vi "McPhersonScan.vi"   [LabVIEW 2019]
types:
  T1 = enum16{"_Quit_", "Init", "Idle", "Error", "BeginScan", "SlewToZ1", "SlewPause", "StartScan", "Scanning", "ScanPause", "FinishScan", "Quit", "BeginSlew", "ResetBacklash"}
  T2 = enum16{"-Slew", "ScanN or SlewN or (Z0=Z1 & FinishScan)", "Error", "Z0=Z1 & BeginScan", "PauseY", "default"}
  T3 = enum16{"ScanN", "Error", "PassZ2", "PauseY", "default"}
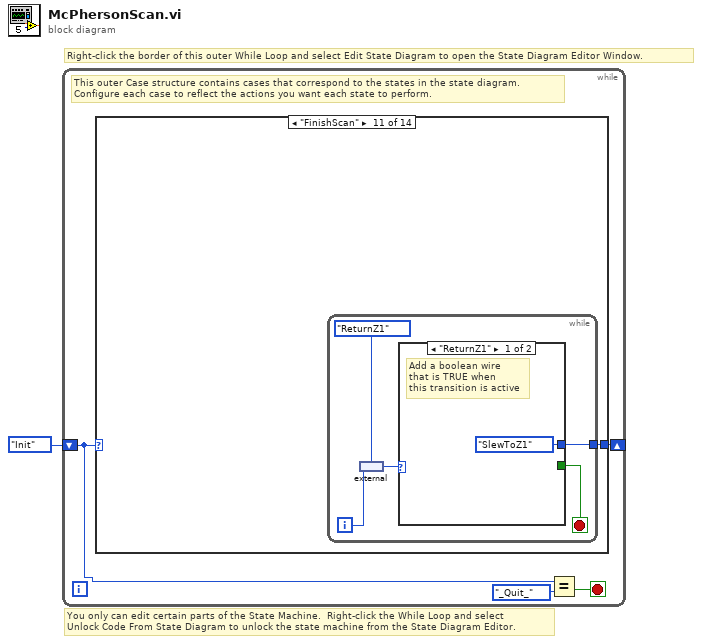
[diagram p0: block diagram]
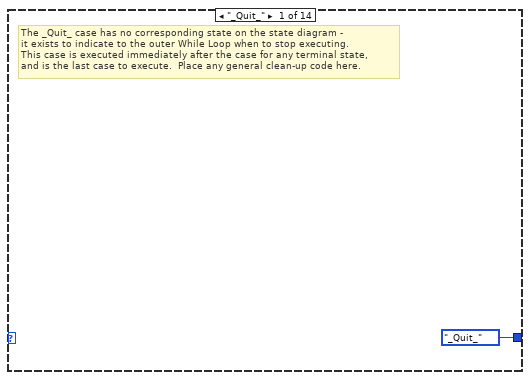
[diagram p2: hidden frame]
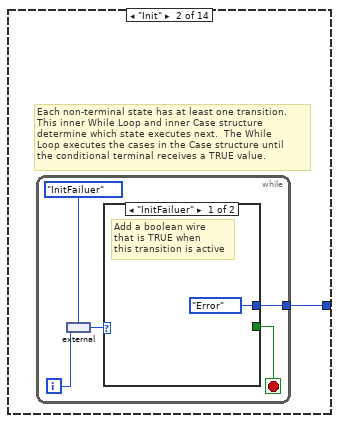
[diagram p3: hidden frame]
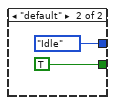
[diagram p4: hidden frame]
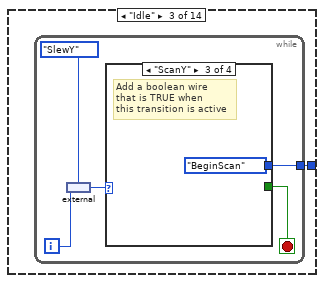
[diagram p5: hidden frame]
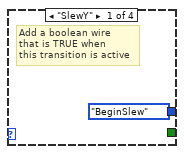
[diagram p6: hidden frame]
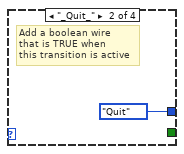
[diagram p7: hidden frame]
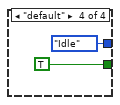
[diagram p8: hidden frame]
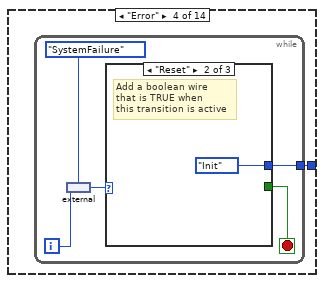
[diagram p9: hidden frame]
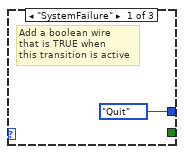
[diagram p10: hidden frame]
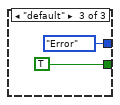
[diagram p11: hidden frame]
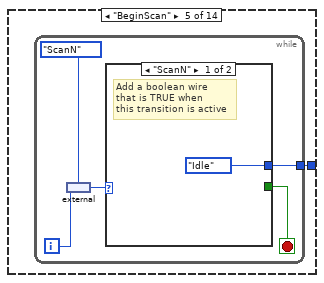
[diagram p12: hidden frame]
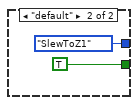
[diagram p13: hidden frame]
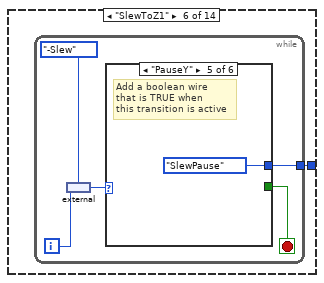
[diagram p14: hidden frame]
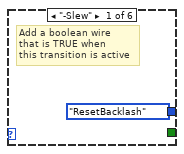
[diagram p15: hidden frame]
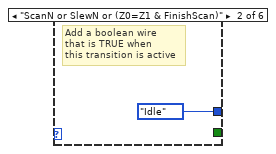
[diagram p16: hidden frame]
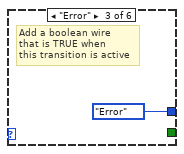
[diagram p17: hidden frame]
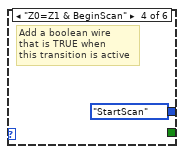
[diagram p18: hidden frame]
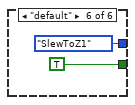
[diagram p19: hidden frame]
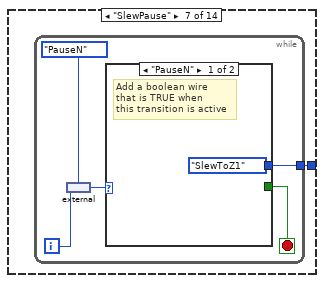
[diagram p20: hidden frame]
diagram:
  # "Right-click the border of this outer While Loop and select Edit State Diagram to open the State Diagram Editor Window."
  # "You only can edit certain parts of the State Machine.  Right-click the While Loop and select \nUnlock Code From State Diagram to unlock the state machine from the State Diagram Editor."
  n1 = while {
    shift-right: [w4] -> _
    shift-left: T1."Init" -> [w5]
    stop <- w3 stop-if-true
    # "This outer Case structure contains cases that correspond to the states in the state diagram.  \nConfigure each case to reflect the actions you want each state to perform."
    n2 = case shown="\"FinishScan\"" w5 {
      tunnel: [T1."_Quit_" w7 w21 w37 w52 w66 w84 w98 w111 w128 w142 w156 w169 w182] -> w4
      frame "_Quit_" {
        # "The _Quit_ case has no corresponding state on the state diagram -\nit exists to indicate to the outer While Loop when to stop executing.\nThis case is executed immediately after the case for any terminal state, \nand is the last case to execute.  Place any general clean-up code here."
      }
      frame "Init" {
        # "Each non-terminal state has at least one transition.\nThis inner While Loop and inner Case structure \ndetermine which state executes next.  The While \nLoop executes the cases in the Case structure until \nthe conditional terminal receives a TRUE value."
        n3 = while {
          tunnel: [w9] -> w7
          i -> [w12]
          stop <- w8 stop-if-true
          n4 = external(enum16{"InitFailuer", "default"}."InitFailuer", w12) -> (w10:enum16{"InitFailuer", "default"})
          n5 = case shown="\"InitFailuer\"" w10 {
            tunnel: [T1."Error" T1."Idle"] -> w9
            tunnel: [_ TRUE] -> w8
            frame "InitFailuer" {
              # "Add a boolean wire\nthat is TRUE when\nthis transition is active"
            }
            frame "default" {
            }
          }
        }
      }
      frame "Idle" {
        n6 = while {
          tunnel: [w23] -> w21
          i -> [w26]
          stop <- w22 stop-if-true
          n7 = external(enum16{"SlewY", "_Quit_", "ScanY", "default"}."SlewY", w26) -> (w24:enum16{"SlewY", "_Quit_", "ScanY", "default"})
          n8 = case shown="\"ScanY\"" w24 {
            tunnel: [T1."BeginSlew" T1."Quit" T1."BeginScan" T1."Idle"] -> w23
            tunnel: [_ _ _ TRUE] -> w22
            frame "SlewY" {
              # "Add a boolean wire\nthat is TRUE when\nthis transition is active"
            }
            frame "_Quit_" {
              # "Add a boolean wire\nthat is TRUE when\nthis transition is active"
            }
            frame "ScanY" {
              # "Add a boolean wire\nthat is TRUE when\nthis transition is active"
            }
            frame "default" {
            }
          }
        }
      }
      frame "Error" {
        n9 = while {
          tunnel: [w39] -> w37
          i -> [w42]
          stop <- w38 stop-if-true
          n10 = external(enum16{"SystemFailure", "Reset", "default"}."SystemFailure", w42) -> (w40:enum16{"SystemFailure", "Reset", "default"})
          n11 = case shown="\"Reset\"" w40 {
            tunnel: [T1."Quit" T1."Init" T1."Error"] -> w39
            tunnel: [_ _ TRUE] -> w38
            frame "SystemFailure" {
              # "Add a boolean wire\nthat is TRUE when\nthis transition is active"
            }
            frame "Reset" {
              # "Add a boolean wire\nthat is TRUE when\nthis transition is active"
            }
            frame "default" {
            }
          }
        }
      }
      frame "BeginScan" {
        n12 = while {
          tunnel: [w54] -> w52
          i -> [w57]
          stop <- w53 stop-if-true
          n13 = external(enum16{"ScanN", "default"}."ScanN", w57) -> (w55:enum16{"ScanN", "default"})
          n14 = case shown="\"ScanN\"" w55 {
            tunnel: [T1."Idle" T1."SlewToZ1"] -> w54
            tunnel: [_ TRUE] -> w53
            frame "ScanN" {
              # "Add a boolean wire\nthat is TRUE when\nthis transition is active"
            }
            frame "default" {
            }
          }
        }
      }
      frame "SlewToZ1" {
        n15 = while {
          tunnel: [w68] -> w66
          i -> [w71]
          stop <- w67 stop-if-true
          n16 = external(T2."-Slew", w71) -> (w69:T2)
          n17 = case shown="\"PauseY\"" w69 {
            tunnel: [T1."ResetBacklash" T1."Idle" T1."Error" T1."StartScan" T1."SlewPause" T1."SlewToZ1"] -> w68
            tunnel: [_ _ _ _ _ TRUE] -> w67
            frame "-Slew" {
              # "Add a boolean wire\nthat is TRUE when\nthis transition is active"
            }
            frame "ScanN or SlewN or (Z0=Z1 & FinishScan)" {
              # "Add a boolean wire\nthat is TRUE when\nthis transition is active"
            }
            frame "Error" {
              # "Add a boolean wire\nthat is TRUE when\nthis transition is active"
            }
            frame "Z0=Z1 & BeginScan" {
              # "Add a boolean wire\nthat is TRUE when\nthis transition is active"
            }
            frame "PauseY" {
              # "Add a boolean wire\nthat is TRUE when\nthis transition is active"
            }
            frame "default" {
            }
          }
        }
      }
      frame "SlewPause" {
        n18 = while {
          tunnel: [w86] -> w84
          i -> [w89]
          stop <- w85 stop-if-true
          n19 = external(enum16{"PauseN", "default"}."PauseN", w89) -> (w87:enum16{"PauseN", "default"})
          n20 = case shown="\"PauseN\"" w87 {
            tunnel: [T1."SlewToZ1" T1."SlewPause"] -> w86
            tunnel: [_ TRUE] -> w85
            frame "PauseN" {
              # "Add a boolean wire\nthat is TRUE when\nthis transition is active"
            }
            frame "default" {
            }
          }
        }
      }
      frame "StartScan" {
        n21 = while {
          tunnel: [w100] -> w98
          i -> [w103]
          stop <- w99 stop-if-true
          n22 = external(enum16{"default"}."default", w103) -> (w101:enum16{"default"})
          n23 = case shown="\"default\"" w101 {
            tunnel: [T1."Scanning"] -> w100
            tunnel: [TRUE] -> w99
            frame "default" {
            }
          }
        }
      }
      frame "Scanning" {
        n24 = while {
          tunnel: [w113] -> w111
          i -> [w116]
          stop <- w112 stop-if-true
          n25 = external(T3."ScanN", w116) -> (w114:T3)
          n26 = case shown="\"PauseY\"" w114 {
            tunnel: [T1."Idle" T1."Error" T1."FinishScan" T1."ScanPause" T1."Scanning"] -> w113
            tunnel: [_ _ _ _ TRUE] -> w112
            frame "ScanN" {
              # "Add a boolean wire\nthat is TRUE when\nthis transition is active"
            }
            frame "Error" {
              # "Add a boolean wire\nthat is TRUE when\nthis transition is active"
            }
            frame "PassZ2" {
              # "Add a boolean wire\nthat is TRUE when\nthis transition is active"
            }
            frame "PauseY" {
              # "Add a boolean wire\nthat is TRUE when\nthis transition is active"
            }
            frame "default" {
            }
          }
        }
      }
      frame "ScanPause" {
        n27 = while {
          tunnel: [w130] -> w128
          i -> [w133]
          stop <- w129 stop-if-true
          n28 = external(enum16{"PauseN", "default"}."PauseN", w133) -> (w131:enum16{"PauseN", "default"})
          n29 = case shown="\"PauseN\"" w131 {
            tunnel: [T1."Scanning" T1."ScanPause"] -> w130
            tunnel: [_ TRUE] -> w129
            frame "PauseN" {
              # "Add a boolean wire\nthat is TRUE when\nthis transition is active"
            }
            frame "default" {
            }
          }
        }
      }
      frame "FinishScan" {
        n30 = while {
          tunnel: [w144] -> w142
          i -> [w147]
          stop <- w143 stop-if-true
          n31 = external(enum16{"ReturnZ1", "default"}."ReturnZ1", w147) -> (w145:enum16{"ReturnZ1", "default"})
          n32 = case shown="\"ReturnZ1\"" w145 {
            tunnel: [T1."SlewToZ1" T1."Idle"] -> w144
            tunnel: [_ TRUE] -> w143
            frame "ReturnZ1" {
              # "Add a boolean wire\nthat is TRUE when\nthis transition is active"
            }
            frame "default" {
            }
          }
        }
      }
      frame "Quit" {
        n33 = while {
          tunnel: [w158] -> w156
          i -> [w161]
          stop <- w157 stop-if-true
          n34 = external(enum16{"default"}."default", w161) -> (w159:enum16{"default"})
          n35 = case shown="\"default\"" w159 {
            tunnel: [T1."Quit"] -> w158
            tunnel: [TRUE] -> w157
            frame "default" {
            }
          }
        }
      }
      frame "BeginSlew" {
        n36 = while {
          tunnel: [w171] -> w169
          i -> [w174]
          stop <- w170 stop-if-true
          n37 = external(enum16{"default"}."default", w174) -> (w172:enum16{"default"})
          n38 = case shown="\"default\"" w172 {
            tunnel: [T1."SlewToZ1"] -> w171
            tunnel: [TRUE] -> w170
            frame "default" {
            }
          }
        }
      }
      frame "ResetBacklash" {
        n39 = while {
          tunnel: [w184] -> w182
          i -> [w187]
          stop <- w183 stop-if-true
          n40 = external(enum16{"default"}."default", w187) -> (w185:enum16{"default"})
          n41 = case shown="\"default\"" w185 {
            tunnel: [T1."Idle"] -> w184
            tunnel: [TRUE] -> w183
            frame "default" {
            }
          }
        }
      }
    }
    n42 = Equal?(x=w5, y=T1."_Quit_") -> (x = y?=w3:bool)
  }
